vi "UDPRead.vi"(8 "connection ID":refnum<k16>, 10 "connection  replay":refnum<k16>, 11 "error in (no error)":errorcluster) -> (0 "Frame":cluster{"ID":u32, "Data":u8[]}[](array[cluster]), 3 "error out":errorcluster)   [LabVIEW 2017]
panel:
  in  "Message length":u16=60
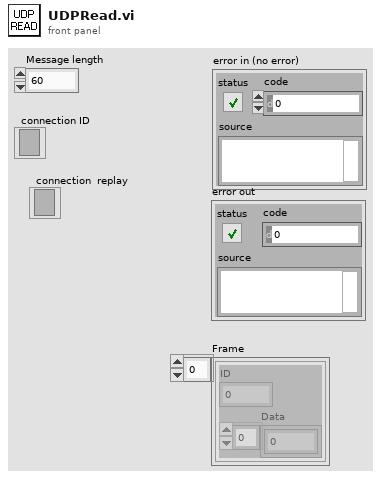
[diagram p1: front panel]
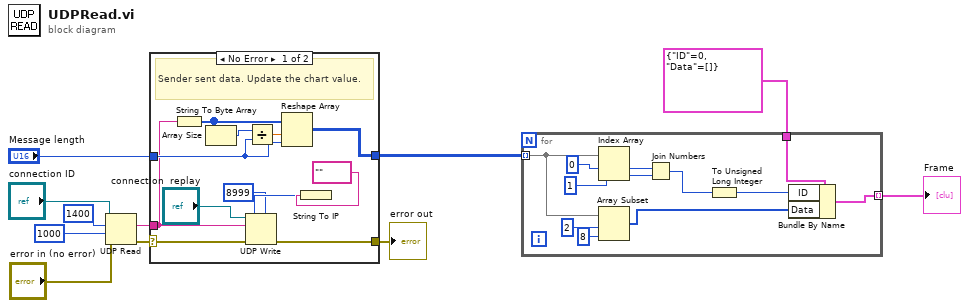
[diagram p0: block diagram]
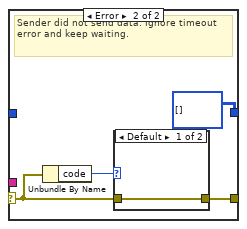
[diagram p2: hidden frame]
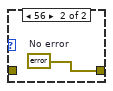
[diagram p3: hidden frame]
diagram:
  n1 = UDP Read(connection ID="connection ID", max size (548)=1400, timeout ms (25000)=1000, 8:"error in (no error)") -> (data out=w1:string, error out=w7:errorcluster)  [unwired: 3 out]
  n2 = case shown="No Error" w7 {
    selector: w7 -> [w16 w26]
    tunnel: w1 -> [w18 _]
    tunnel: [w15 w25] -> w3
    tunnel: [w20 u8[][] [] ("unsigned byte array")] -> w2
    tunnel: "Message length" -> [w19 _]
    frame No Error {
      # "Sender sent data. Update the chart value."
      n3 = String To Byte Array(string=w18) -> (unsigned byte array=w23:u8[])
      n4 = Array Size(array=w23) -> (size(s)=w22:i32)
      n5 = Divide(x=w22, y=w19) -> (x/y=w21:dbl)
      n6 = Reshape Array(w23, w21, w19) -> (w20:u8[][])
      n7 = String To IP(1:"") -> (0:w13:u32)
      n8 = UDP Write(address=w13, port or service name=u16 8999, connection ID="connection  replay", data in=w18, 8:w16) -> (error out=w15:errorcluster)  [unwired: 1 in, 1 out]
    }
    frame Error {
      # "Sender did not send data. Ignore timeout error and keep waiting."
      n9 = Unbundle By Name(w26) -> ("code"=w27:i32)
      n10 = case shown="Default" w27 {
        tunnel: w26 -> [w28 _]
        tunnel: [w28 w29] -> w25
        frame Default {
        }
        frame 56 {
          w29 = errorcluster {"status"=FALSE, "code"=0, "source"=""}  # No error
        }
      }
    }
  }
  "error out" <- w3
  n11 = for {
    tunnel: cluster{"ID":u32, "Data":u8[]} {"ID"=0, "Data"=[]} -> [w41]
    tunnel: [w40] -> w10 mode=indexing
    tunnel: w2 -> [w35] mode=indexing
    n12 = Index Array(array=w35, index #1=0 ("index"), index #2=1 ("index")) -> (element #1=w39:u8, element #2=w38:u8)
    n13 = Array Subset(array=w35, index=2, length=8) -> (w33:u8[])
    n14 = Join Numbers(hi=w39, lo=w38) -> ((hi.lo)=w32:u16)
    n15 = To Unsigned Long Integer(number=w32) -> (unsigned 32bit integer=w31:u32)
    n16 = Bundle By Name(cluster=w41, "ID"=w31, "Data"=w33) -> (w40:cluster{"ID":u32, "Data":u8[]})
  }
  "Frame" <- w10
